vi "close in rte.vi"(11 "caller VI":refnum<vi>) -> ()   [LabVIEW 2013, in "NISE Tools VI Server.lvlib"]
uses:
  NISE Tools VI Server.lvlib
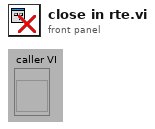
[diagram p1: front panel]
types:
  T1 = enum32{"invalid app kind", "Development System", "Run Time System", "Student Edition", "Embedded LabVIEW", "Evaluation", "Custom"}
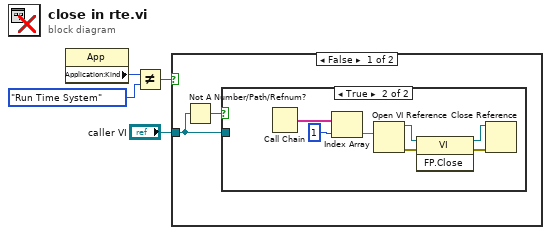
[diagram p0: block diagram]
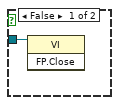
[diagram p2: hidden frame]
diagram:
  n1 = property class="App"() -> ("Application:Kind"=w2:T1)  [unwired: 2 in, 2 out]
  n2 = Not Equal?(x=w2, y=T1."Run Time System" ("Application:Kind")) -> (x != y?=w3:bool)
  n3 = case shown="False" w3 {
    tunnel: "caller VI" -> [w5 _]
    frame False {
      n4 = Not A Number/Path/Refnum?(number/path/refnum=w5) -> (NaN/Path/Refnum?=w6:bool)
      n5 = case shown="True" w6 {
        tunnel: w5 -> [w7 _]
        frame False {
          n6 = invoke class="VI" method="FP.Close"(reference=w7) -> ()  [unwired: 2 in, 3 out]
        }
        frame True {
          n7 = Call Chain() -> (call chain=w14:string[])
          n8 = Index Array(array=w14, index=1) -> (element=w12:string)
          n9 = Open VI Reference(vi path=w12) -> (vi reference=w9:refnum<vi>, error out=w11:errorcluster)  [unwired: 5 in]
          n10 = invoke class="VI" method="FP.Close"(reference=w9, error in=w11) -> (reference out=w8:refnum<vi>, error out=w10:errorcluster)  [unwired: 1 in, 1 out]
          n11 = Close Reference(reference=w8, error in (no error)=w10) -> ()  [unwired: 1 out]
        }
      }
    }
    frame True {
    }
  }
